vi "Input data row.vi"(8 "error in (no error)":errorcluster, 11 "Automatic Mode in":refnum<class "Automatic Mode.lvclass">) -> (0 "error out":errorcluster, 3 "Automatic Mode out":refnum<class "Automatic Mode.lvclass">)   [LabVIEW 2015, in "Automatic Mode.lvclass"]
uses:
  Automatic Mode.lvclass
panel:
  in  "Last row of data file":string[](array[string])
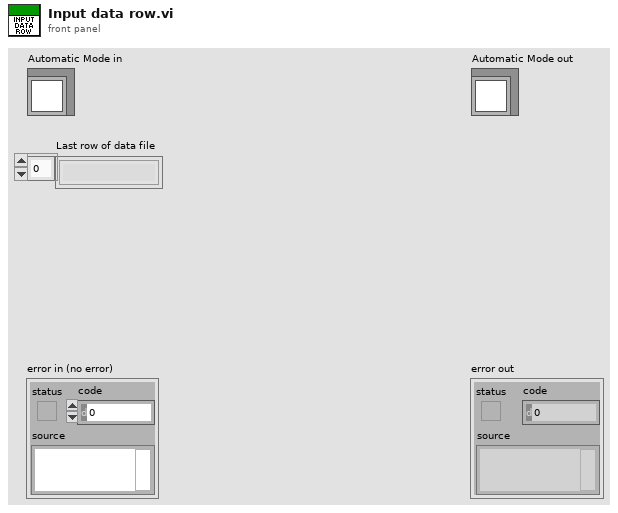
[diagram p1: front panel]
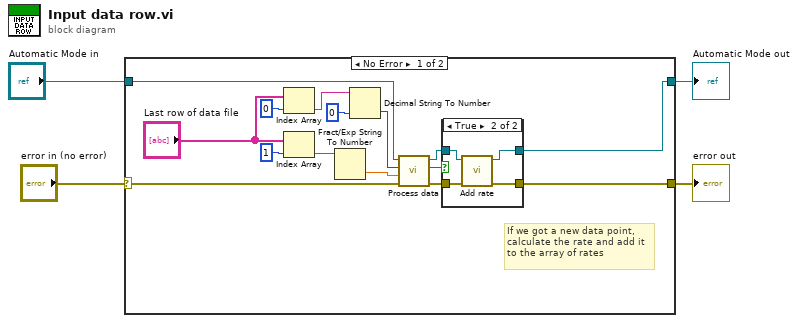
[diagram p0: block diagram]
diagram:
  n1 = case shown="No Error" "error in (no error)" {
    selector: "error in (no error)" -> [w10 w27]
    tunnel: [w5 w27] -> w3
    tunnel: [w6 w26] -> w1
    tunnel: "Automatic Mode in" -> [w13 w26]
    frame No Error {
      # "If we got a new data point,\ncalculate the rate and add it\nto the array of rates"
      n2 = Index Array(array="Last row of data file", index=0) -> (element=w17:string)
      n3 = Index Array(array="Last row of data file", index=1) -> (element=w16:string)
      n4 = Fract/Exp String To Number(string=w16) -> (number=w11:dbl)  [unwired: 3 in, 1 out]
      n5 = Decimal String To Number(string=w17, default (0L)=i64 0 ("default (0 I32)")) -> (number=w12:i64)  [unwired: 1 in, 1 out]
      n6 = call "Process data.vi"("error in (no error)"=w10, "New polarization"=w11, "New eventnum"=w12, "Automatic Mode in"=w13) -> ("error out"=w7:errorcluster, "Added new data point?"=w9:bool, "Automatic Mode out"=w8:refnum<class "Automatic Mode.lvclass">)  [unwired: 5 in]
      n7 = case shown="True" w9 {
        tunnel: w8 -> [w21 w25]
        tunnel: w7 -> [w20 w24]
        tunnel: [w21 w23] -> w6
        tunnel: [w20 w22] -> w5
        frame False {
        }
        frame True {
          n8 = call "Add rate.vi"("error in (no error)"=w24, "Automatic Mode in"=w25) -> ("error out"=w22:errorcluster, "Automatic Mode out"=w23:refnum<class "Automatic Mode.lvclass">)  [unwired: 8 in]
        }
      }
    }
    frame Error {
    }
  }
  "error out" <- w3
  "Automatic Mode out" <- w1
